vi "Do.vi"(8 "error in (no error)":errorcluster, 10 "Actor in":refnum<class "Actor.lvclass">, 11 "Send Message to Nested Actor Msg":refnum<class "Fwd Message to Nested Actor Msg.lvclass">) -> (0 "error out":errorcluster, 2 "Actor out":refnum<class "Actor.lvclass">)   [LabVIEW 2023, in "Coffee Shop.lvlib" / "Fwd Message to Nested Actor Msg.lvclass"]
doc: "This VI delivers the message to the actor by calling the appropriate method(s) on the actor."
uses:
  Fwd Message to Nested Actor Msg.lvclass
  <vilib>/ActorFramework/Actor/Actor.lvclass
  Coffee Shop/Coffee Shop.lvclass
  c:/dev/_r/4/eng/lv-core/lvpostprocessingd/lv_mc_x86_64/dist_i386/vi.lib/ActorFramework/Actor/Actor.lvclass
  Fwd Message to Nested Actor Msg.lvclass/Fwd Message to Nested Actor Msg.ctl
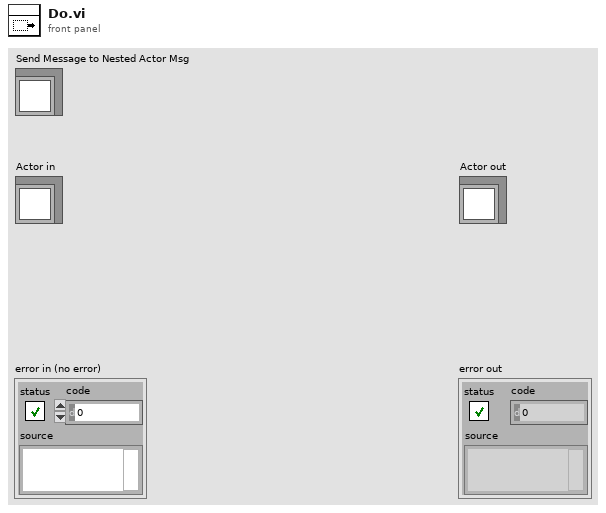
[diagram p1: front panel]
types:
  T1 = typedef "Coffee Shop.lvlib/Coffee Shop.lvclass/Entity Types.ctl" = enum16{"Customer", "Cashier", "Barista"}
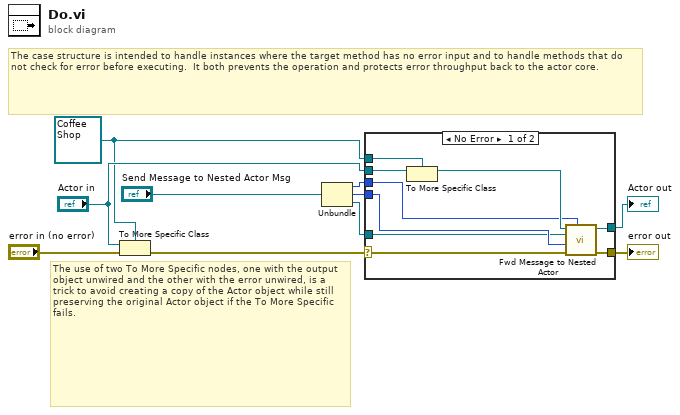
[diagram p0: block diagram]
diagram:
  w4 = refnum<class "Coffee Shop.lvclass"> refnum ("Actor in")
  # "The use of two To More Specific nodes, one with the output object unwired and the other with the error unwired, is a trick to avoid creating a copy of the Actor object while still preserving the original Actor object if the To More Specific fails."
  # "The case structure is intended to handle instances where the target method has no error input and to handle methods that do not check for error before executing.  It both prevents the operation and protects error throughput back to the actor core."
  n1 = To More Specific Class(target class=w4, reference="Actor in", error in="error in (no error)") -> (error out=w8:errorcluster)  [unwired: 1 out]
  n2 = Unbundle("Send Message to Nested Actor Msg") -> (w3:T1, w2:i32, w1:refnum<class "Message.lvclass">)
  n3 = case shown="No Error" w8 {
    selector: w8 -> [w17 w21]
    tunnel: [w19 w21] -> w7
    tunnel: [w18 w20] -> w6
    tunnel: "Actor in" -> [w16 w20]
    tunnel: w4 -> [w15 _]
    tunnel: w3 -> [w11 _]
    tunnel: w2 -> [w13 _]
    tunnel: w1 -> [w12 _]
    frame No Error {
      n4 = To More Specific Class(target class=w15, reference=w16) -> (specific class reference=w14:refnum<class "Coffee Shop.lvclass">)  [unwired: 1 in, 1 out]
      n5 = call-dynamic "Fwd Message to Nested Actor.vi"("Entity Type"=w11, "error in (no error)"=w17, "Entity Index"=w13, "Message"=w12, "Coffee Shop in"=w14) -> ("error out"=w19:errorcluster, "Coffee Shop out"=w18:refnum<class "Coffee Shop.lvclass">)  [unwired: 5 in]
    }
    frame Error {
      # "If type check fails, pass the original object out again."
    }
  }
  "error out" <- w7
  "Actor out" <- w6
